vi "ManualPeopleCounting.vi"() -> ()   [LabVIEW 2011]
panel:
  in  "Note 0":string="N"
  in  "0":bool
  in  "Note -3+1":string="N"
  in  "Note +3-1":string="N"
  in  "-3+1":bool
  in  "+3-1":bool
  in  "Note -2+1":string="N"
  in  "Note +2-1":string="N"
  in  "-2+1":bool
  in  "+2-1":bool
  in  "Note -5":string="N"
  in  "- 5":bool
  in  "+5":bool
  in  "Note +5":string="N"
  in  "Note -4":string="N"
  in  "- 4":bool
  in  "+ 4":bool
  in  "Note +4":string="N"
  in  "-999":bool
  in  "Note -999":string="GoOut"
  in  "Note 999":string="N"
  in  "Note -1+1":string="N"
  in  "Note +-1":string="N"
  in  "Note -3":string="N"
  in  "Note +3":string="N"
  in  "Note -2":string="N"
  in  "Note +2":string="N"
  in  "999":bool
  in  "-1+1":bool
  in  "- 3":bool
  in  "+1-1":bool
  in  "+3":bool
  in  "- 2":bool
  in  "+2":bool
  in  "-1":bool
  in  "Note -1":string="N"
  in  "Note +1":string="N"
  in  "+1":bool
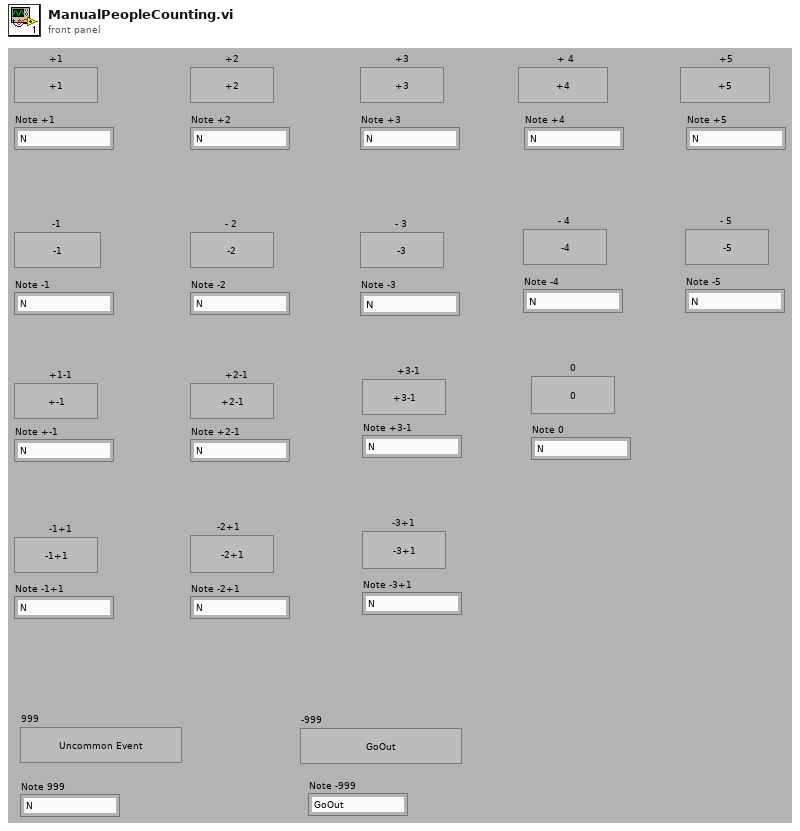
[diagram p1: front panel]
types:
  T1 = enum16{"open", "replace", "create", "open or create", "replace or create", "replace or create with confirmation"}
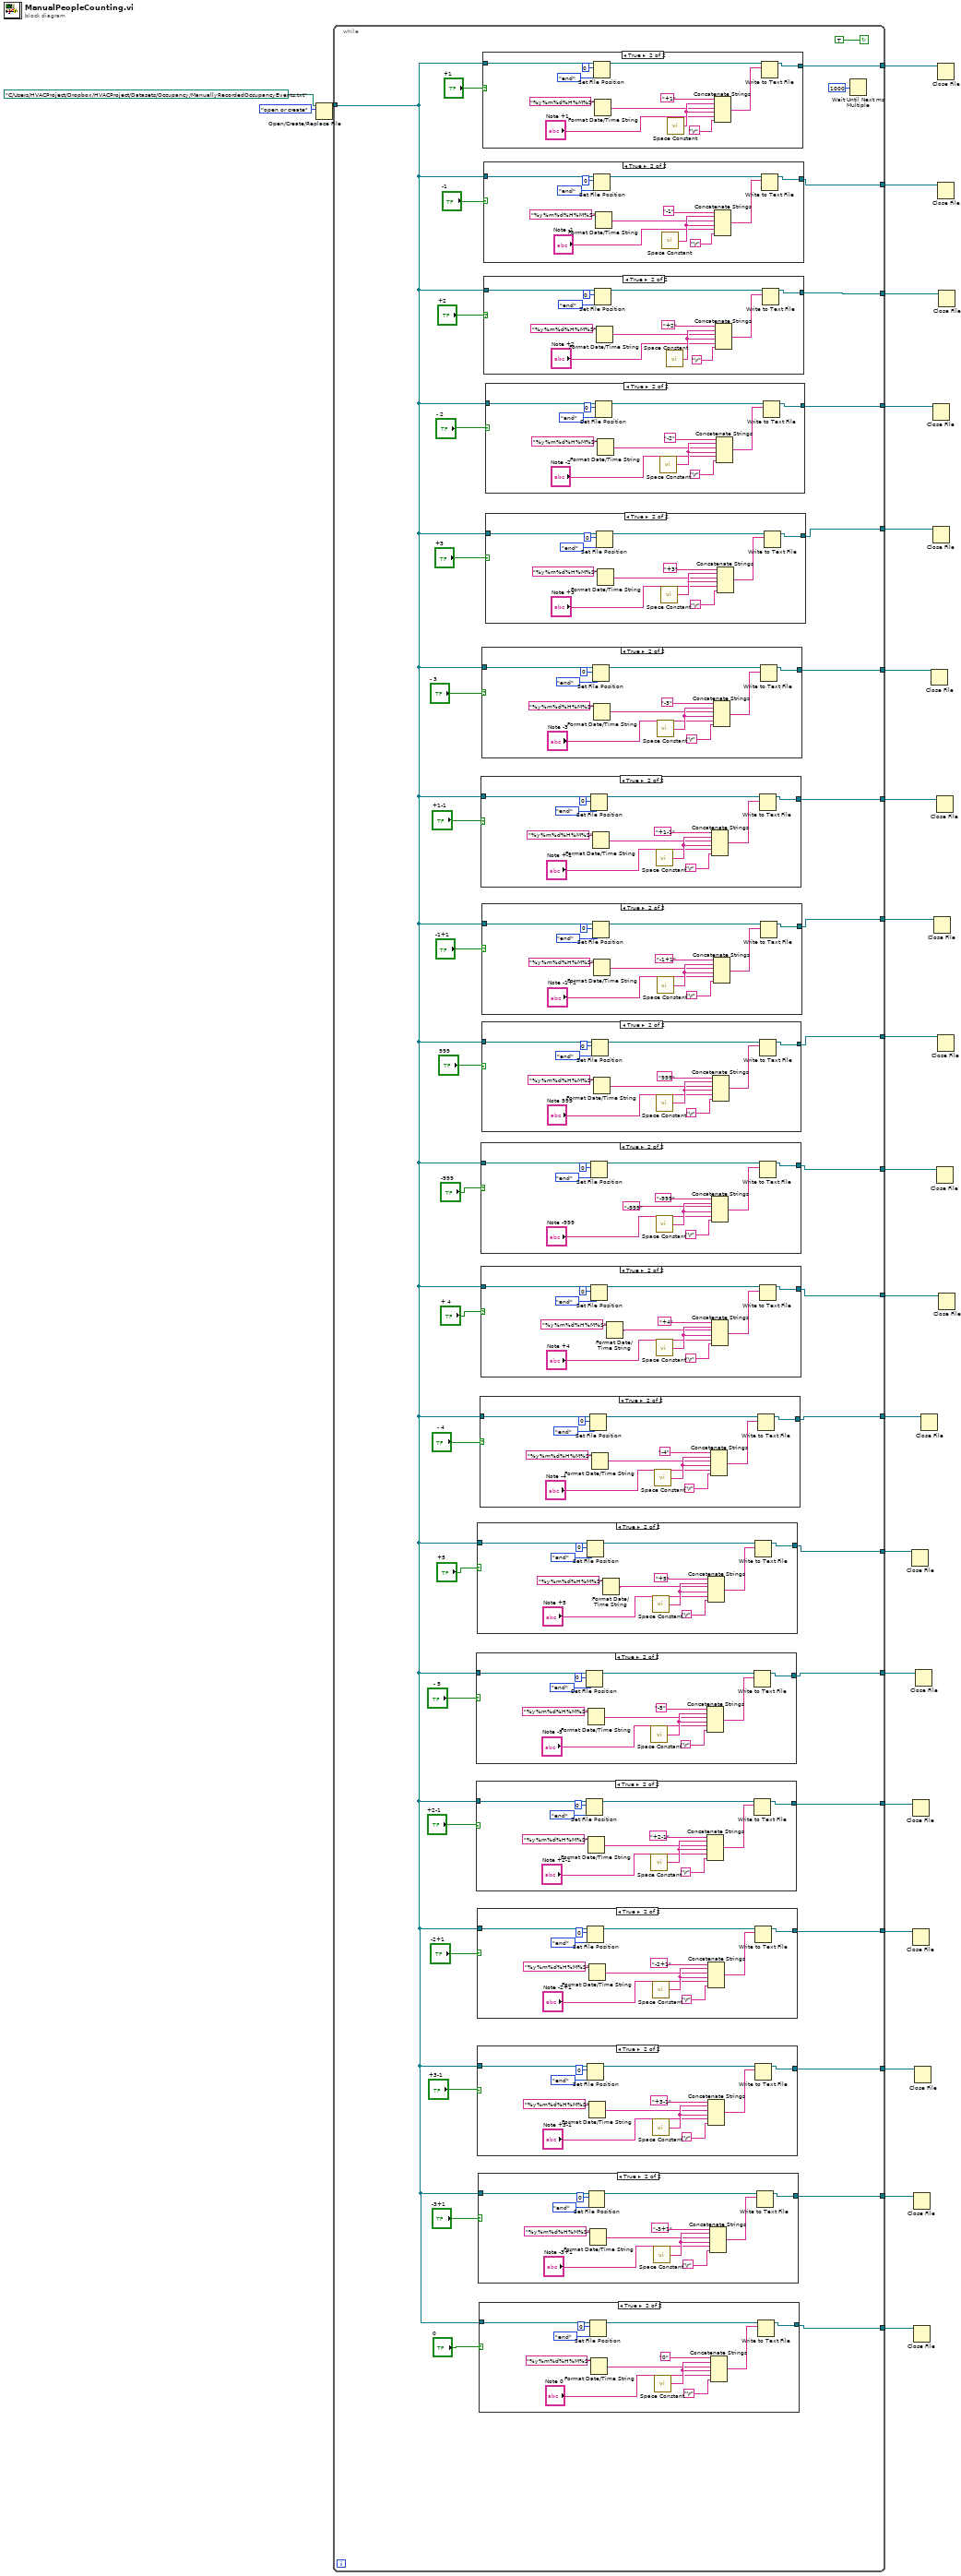
[diagram p0: block diagram]
diagram:
  n1 = Open/Create/Replace File(file path (use dialog)=path "C:/Users/HVACProject/Dropbox/HVACProject/Datasets/Occupancy/ManuallyRecordedOccupancyEvents.txt" ("file (use dialog)"), operation (0:open)=T1."open or create") -> (refnum out=w20:refnum<file>)  [unwired: 4 in, 2 out]
  n2 = while {
    tunnel: w20 -> [w24]
    tunnel: [w59] -> w19
    tunnel: [w58] -> w18
    tunnel: [w56] -> w17
    tunnel: [w54] -> w16
    tunnel: [w52] -> w15
    tunnel: [w50] -> w14
    tunnel: [w48] -> w13
    tunnel: [w46] -> w12
    tunnel: [w44] -> w11
    tunnel: [w43] -> w10
    tunnel: [w40] -> w9
    tunnel: [w38] -> w8
    tunnel: [w35] -> w7
    tunnel: [w34] -> w6
    tunnel: [w31] -> w5
    tunnel: [w30] -> w4
    tunnel: [w27] -> w3
    tunnel: [w26] -> w2
    tunnel: [w23] -> w1
    stop <- TRUE continue-if-true
    n3 = case shown="True" "- 5" {
      tunnel: [w129 w131] -> w35
      tunnel: w24 -> [w129 w141]
      frame False {
      }
      frame True {
        n4 = Set File Position(offset (in bytes) (0)=i64 0, refnum=w141, from (0:start)=enum16{"start", "end", "current"}."end") -> (refnum out=w138:refnum<file>)  [unwired: 1 in, 1 out]
        n5 = Format Date/Time String(time format string (%c)="%y%m%d%H%M%S") -> (date/time string=w133:string)  [unwired: 2 in]
        n6 = call <vilib>:"Space Constant.vi"() -> ("String"=w135:string)
        n7 = Concatenate Strings("-5" ("string"), w135, w133, w135, "Note -5", "\r") -> (w137:string)
        n8 = Write to Text File(file (use dialog)=w138, text=w137) -> (refnum out=w131:refnum<file>)  [unwired: 2 in, 2 out]
      }
    }
    n9 = case shown="True" "+2-1" {
      tunnel: [w116 w118] -> w31
      tunnel: w24 -> [w116 w128]
      frame False {
      }
      frame True {
        n10 = Set File Position(offset (in bytes) (0)=i64 0, refnum=w128, from (0:start)=enum16{"start", "end", "current"}."end") -> (refnum out=w125:refnum<file>)  [unwired: 1 in, 1 out]
        n11 = Format Date/Time String(time format string (%c)="%y%m%d%H%M%S") -> (date/time string=w120:string)  [unwired: 2 in]
        n12 = call <vilib>:"Space Constant.vi"() -> ("String"=w122:string)
        n13 = Concatenate Strings("+2-1" ("string"), w122, w120, w122, "Note +2-1", "\r") -> (w124:string)
        n14 = Write to Text File(file (use dialog)=w125, text=w124) -> (refnum out=w118:refnum<file>)  [unwired: 2 in, 2 out]
      }
    }
    n15 = case shown="True" "+5" {
      tunnel: [w142 w146] -> w34
      tunnel: w24 -> [w142 w154]
      frame False {
      }
      frame True {
        n16 = Set File Position(offset (in bytes) (0)=i64 0, refnum=w154, from (0:start)=enum16{"start", "end", "current"}."end") -> (refnum out=w151:refnum<file>)  [unwired: 1 in, 1 out]
        n17 = Format Date/Time String(time format string (%c)="%y%m%d%H%M%S") -> (date/time string=w143:string)  [unwired: 2 in]
        n18 = call <vilib>:"Space Constant.vi"() -> ("String"=w148:string)
        n19 = Concatenate Strings("+5" ("string"), w148, w143, w148, "Note +5", "\r") -> (w150:string)
        n20 = Write to Text File(file (use dialog)=w151, text=w150) -> (refnum out=w146:refnum<file>)  [unwired: 2 in, 2 out]
      }
    }
    n21 = case shown="True" "-2+1" {
      tunnel: [w103 w105] -> w30
      tunnel: w24 -> [w103 w115]
      frame False {
      }
      frame True {
        n22 = Set File Position(offset (in bytes) (0)=i64 0, refnum=w115, from (0:start)=enum16{"start", "end", "current"}."end") -> (refnum out=w112:refnum<file>)  [unwired: 1 in, 1 out]
        n23 = Format Date/Time String(time format string (%c)="%y%m%d%H%M%S") -> (date/time string=w107:string)  [unwired: 2 in]
        n24 = call <vilib>:"Space Constant.vi"() -> ("String"=w109:string)
        n25 = Concatenate Strings("-2+1" ("string"), w109, w107, w109, "Note -2+1", "\r") -> (w111:string)
        n26 = Write to Text File(file (use dialog)=w112, text=w111) -> (refnum out=w105:refnum<file>)  [unwired: 2 in, 2 out]
      }
    }
    n27 = case shown="True" "+3-1" {
      tunnel: [w90 w92] -> w27
      tunnel: w24 -> [w90 w102]
      frame False {
      }
      frame True {
        n28 = Set File Position(offset (in bytes) (0)=i64 0, refnum=w102, from (0:start)=enum16{"start", "end", "current"}."end") -> (refnum out=w99:refnum<file>)  [unwired: 1 in, 1 out]
        n29 = Format Date/Time String(time format string (%c)="%y%m%d%H%M%S") -> (date/time string=w94:string)  [unwired: 2 in]
        n30 = call <vilib>:"Space Constant.vi"() -> ("String"=w96:string)
        n31 = Concatenate Strings("+3-1" ("string"), w96, w94, w96, "Note +3-1", "\r") -> (w98:string)
        n32 = Write to Text File(file (use dialog)=w99, text=w98) -> (refnum out=w92:refnum<file>)  [unwired: 2 in, 2 out]
      }
    }
    n33 = case shown="True" "-3+1" {
      tunnel: [w77 w79] -> w26
      tunnel: w24 -> [w77 w89]
      frame False {
      }
      frame True {
        n34 = Set File Position(offset (in bytes) (0)=i64 0, refnum=w89, from (0:start)=enum16{"start", "end", "current"}."end") -> (refnum out=w86:refnum<file>)  [unwired: 1 in, 1 out]
        n35 = Format Date/Time String(time format string (%c)="%y%m%d%H%M%S") -> (date/time string=w81:string)  [unwired: 2 in]
        n36 = call <vilib>:"Space Constant.vi"() -> ("String"=w83:string)
        n37 = Concatenate Strings("-3+1" ("string"), w83, w81, w83, "Note -3+1", "\r") -> (w85:string)
        n38 = Write to Text File(file (use dialog)=w86, text=w85) -> (refnum out=w79:refnum<file>)  [unwired: 2 in, 2 out]
      }
    }
    n39 = case shown="True" "0" {
      tunnel: [w64 w66] -> w23
      tunnel: w24 -> [w64 w76]
      frame False {
      }
      frame True {
        n40 = Set File Position(offset (in bytes) (0)=i64 0, refnum=w76, from (0:start)=enum16{"start", "end", "current"}."end") -> (refnum out=w73:refnum<file>)  [unwired: 1 in, 1 out]
        n41 = Format Date/Time String(time format string (%c)="%y%m%d%H%M%S") -> (date/time string=w68:string)  [unwired: 2 in]
        n42 = call <vilib>:"Space Constant.vi"() -> ("String"=w70:string)
        n43 = Concatenate Strings("0" ("string"), w70, w68, w70, "Note 0", "\r") -> (w72:string)
        n44 = Write to Text File(file (use dialog)=w73, text=w72) -> (refnum out=w66:refnum<file>)  [unwired: 2 in, 2 out]
      }
    }
    n45 = case shown="True" "- 4" {
      tunnel: [w155 w157] -> w38
      tunnel: w24 -> [w155 w167]
      frame False {
      }
      frame True {
        n46 = Set File Position(offset (in bytes) (0)=i64 0, refnum=w167, from (0:start)=enum16{"start", "end", "current"}."end") -> (refnum out=w164:refnum<file>)  [unwired: 1 in, 1 out]
        n47 = Format Date/Time String(time format string (%c)="%y%m%d%H%M%S") -> (date/time string=w159:string)  [unwired: 2 in]
        n48 = call <vilib>:"Space Constant.vi"() -> ("String"=w161:string)
        n49 = Concatenate Strings("-4" ("string"), w161, w159, w161, "Note -4", "\r") -> (w163:string)
        n50 = Write to Text File(file (use dialog)=w164, text=w163) -> (refnum out=w157:refnum<file>)  [unwired: 2 in, 2 out]
      }
    }
    n51 = case shown="True" "+1-1" {
      tunnel: [w219 w221] -> w48
      tunnel: w24 -> [w219 w231]
      frame False {
      }
      frame True {
        n52 = Set File Position(offset (in bytes) (0)=i64 0, refnum=w231, from (0:start)=enum16{"start", "end", "current"}."end") -> (refnum out=w228:refnum<file>)  [unwired: 1 in, 1 out]
        n53 = Format Date/Time String(time format string (%c)="%y%m%d%H%M%S") -> (date/time string=w223:string)  [unwired: 2 in]
        n54 = call <vilib>:"Space Constant.vi"() -> ("String"=w225:string)
        n55 = Concatenate Strings("+1-1" ("string"), w225, w223, w225, "Note +-1", "\r") -> (w227:string)
        n56 = Write to Text File(file (use dialog)=w228, text=w227) -> (refnum out=w221:refnum<file>)  [unwired: 2 in, 2 out]
      }
    }
    n57 = case shown="True" "-999" {
      tunnel: [w181 w184] -> w43
      tunnel: w24 -> [w181 w192]
      frame False {
      }
      frame True {
        n58 = Set File Position(offset (in bytes) (0)=i64 0, refnum=w192, from (0:start)=enum16{"start", "end", "current"}."end") -> (refnum out=w189:refnum<file>)  [unwired: 1 in, 1 out]
        n59 = call <vilib>:"Space Constant.vi"() -> ("String"=w186:string)
        n60 = Concatenate Strings("-999" ("string"), w186, "-999" ("string"), w186, "Note -999", "\r") -> (w188:string)
        n61 = Write to Text File(file (use dialog)=w189, text=w188) -> (refnum out=w184:refnum<file>)  [unwired: 2 in, 2 out]
      }
    }
    n62 = case shown="True" "+ 4" {
      tunnel: [w168 w172] -> w40
      tunnel: w24 -> [w168 w180]
      frame False {
      }
      frame True {
        n63 = Set File Position(offset (in bytes) (0)=i64 0, refnum=w180, from (0:start)=enum16{"start", "end", "current"}."end") -> (refnum out=w177:refnum<file>)  [unwired: 1 in, 1 out]
        n64 = Format Date/Time String(time format string (%c)="%y%m%d%H%M%S") -> (date/time string=w169:string)  [unwired: 2 in]
        n65 = call <vilib>:"Space Constant.vi"() -> ("String"=w174:string)
        n66 = Concatenate Strings("+4" ("string"), w174, w169, w174, "Note +4", "\r") -> (w176:string)
        n67 = Write to Text File(file (use dialog)=w177, text=w176) -> (refnum out=w172:refnum<file>)  [unwired: 2 in, 2 out]
      }
    }
    n68 = case shown="True" "999" {
      tunnel: [w193 w195] -> w44
      tunnel: w24 -> [w193 w205]
      frame False {
      }
      frame True {
        n69 = Set File Position(offset (in bytes) (0)=i64 0, refnum=w205, from (0:start)=enum16{"start", "end", "current"}."end") -> (refnum out=w202:refnum<file>)  [unwired: 1 in, 1 out]
        n70 = Format Date/Time String(time format string (%c)="%y%m%d%H%M%S") -> (date/time string=w197:string)  [unwired: 2 in]
        n71 = call <vilib>:"Space Constant.vi"() -> ("String"=w199:string)
        n72 = Concatenate Strings("999" ("string"), w199, w197, w199, "Note 999", "\r") -> (w201:string)
        n73 = Write to Text File(file (use dialog)=w202, text=w201) -> (refnum out=w195:refnum<file>)  [unwired: 2 in, 2 out]
      }
    }
    n74 = case shown="True" "- 3" {
      tunnel: [w232 w234] -> w50
      tunnel: w24 -> [w232 w244]
      frame False {
      }
      frame True {
        n75 = Set File Position(offset (in bytes) (0)=i64 0, refnum=w244, from (0:start)=enum16{"start", "end", "current"}."end") -> (refnum out=w241:refnum<file>)  [unwired: 1 in, 1 out]
        n76 = Format Date/Time String(time format string (%c)="%y%m%d%H%M%S") -> (date/time string=w236:string)  [unwired: 2 in]
        n77 = call <vilib>:"Space Constant.vi"() -> ("String"=w238:string)
        n78 = Concatenate Strings("-3" ("string"), w238, w236, w238, "Note -3", "\r") -> (w240:string)
        n79 = Write to Text File(file (use dialog)=w241, text=w240) -> (refnum out=w234:refnum<file>)  [unwired: 2 in, 2 out]
      }
    }
    n80 = case shown="True" "-1+1" {
      tunnel: [w206 w208] -> w46
      tunnel: w24 -> [w206 w218]
      frame False {
      }
      frame True {
        n81 = Set File Position(offset (in bytes) (0)=i64 0, refnum=w218, from (0:start)=enum16{"start", "end", "current"}."end") -> (refnum out=w215:refnum<file>)  [unwired: 1 in, 1 out]
        n82 = Format Date/Time String(time format string (%c)="%y%m%d%H%M%S") -> (date/time string=w210:string)  [unwired: 2 in]
        n83 = call <vilib>:"Space Constant.vi"() -> ("String"=w212:string)
        n84 = Concatenate Strings("-1+1" ("string"), w212, w210, w212, "Note -1+1", "\r") -> (w214:string)
        n85 = Write to Text File(file (use dialog)=w215, text=w214) -> (refnum out=w208:refnum<file>)  [unwired: 2 in, 2 out]
      }
    }
    n86 = case shown="True" "+1" {
      tunnel: [w297 w299] -> w59
      tunnel: w24 -> [w297 w309]
      frame False {
      }
      frame True {
        n87 = Set File Position(offset (in bytes) (0)=i64 0, refnum=w309, from (0:start)=enum16{"start", "end", "current"}."end") -> (refnum out=w306:refnum<file>)  [unwired: 1 in, 1 out]
        n88 = Format Date/Time String(time format string (%c)="%y%m%d%H%M%S") -> (date/time string=w301:string)  [unwired: 2 in]
        n89 = call <vilib>:"Space Constant.vi"() -> ("String"=w303:string)
        n90 = Concatenate Strings("+1" ("string"), w303, w301, w303, "Note +1", "\r") -> (w305:string)
        n91 = Write to Text File(file (use dialog)=w306, text=w305) -> (refnum out=w299:refnum<file>)  [unwired: 2 in, 2 out]
      }
    }
    n92 = case shown="True" "-1" {
      tunnel: [w284 w286] -> w58
      tunnel: w24 -> [w284 w296]
      frame False {
      }
      frame True {
        n93 = Set File Position(offset (in bytes) (0)=i64 0, refnum=w296, from (0:start)=enum16{"start", "end", "current"}."end") -> (refnum out=w293:refnum<file>)  [unwired: 1 in, 1 out]
        n94 = Format Date/Time String(time format string (%c)="%y%m%d%H%M%S") -> (date/time string=w288:string)  [unwired: 2 in]
        n95 = call <vilib>:"Space Constant.vi"() -> ("String"=w290:string)
        n96 = Concatenate Strings("-1" ("string"), w290, w288, w290, "Note -1", "\r") -> (w292:string)
        n97 = Write to Text File(file (use dialog)=w293, text=w292) -> (refnum out=w286:refnum<file>)  [unwired: 2 in, 2 out]
      }
    }
    n98 = case shown="True" "+2" {
      tunnel: [w271 w273] -> w56
      tunnel: w24 -> [w271 w283]
      frame False {
      }
      frame True {
        n99 = Set File Position(offset (in bytes) (0)=i64 0, refnum=w283, from (0:start)=enum16{"start", "end", "current"}."end") -> (refnum out=w280:refnum<file>)  [unwired: 1 in, 1 out]
        n100 = Format Date/Time String(time format string (%c)="%y%m%d%H%M%S") -> (date/time string=w275:string)  [unwired: 2 in]
        n101 = call <vilib>:"Space Constant.vi"() -> ("String"=w277:string)
        n102 = Concatenate Strings("+2" ("string"), w277, w275, w277, "Note +2", "\r") -> (w279:string)
        n103 = Write to Text File(file (use dialog)=w280, text=w279) -> (refnum out=w273:refnum<file>)  [unwired: 2 in, 2 out]
      }
    }
    n104 = case shown="True" "- 2" {
      tunnel: [w258 w260] -> w54
      tunnel: w24 -> [w258 w270]
      frame False {
      }
      frame True {
        n105 = Set File Position(offset (in bytes) (0)=i64 0, refnum=w270, from (0:start)=enum16{"start", "end", "current"}."end") -> (refnum out=w267:refnum<file>)  [unwired: 1 in, 1 out]
        n106 = Format Date/Time String(time format string (%c)="%y%m%d%H%M%S") -> (date/time string=w262:string)  [unwired: 2 in]
        n107 = call <vilib>:"Space Constant.vi"() -> ("String"=w264:string)
        n108 = Concatenate Strings("-2" ("string"), w264, w262, w264, "Note -2", "\r") -> (w266:string)
        n109 = Write to Text File(file (use dialog)=w267, text=w266) -> (refnum out=w260:refnum<file>)  [unwired: 2 in, 2 out]
      }
    }
    n110 = case shown="True" "+3" {
      tunnel: [w245 w247] -> w52
      tunnel: w24 -> [w245 w257]
      frame False {
      }
      frame True {
        n111 = Set File Position(offset (in bytes) (0)=i64 0, refnum=w257, from (0:start)=enum16{"start", "end", "current"}."end") -> (refnum out=w254:refnum<file>)  [unwired: 1 in, 1 out]
        n112 = Format Date/Time String(time format string (%c)="%y%m%d%H%M%S") -> (date/time string=w249:string)  [unwired: 2 in]
        n113 = call <vilib>:"Space Constant.vi"() -> ("String"=w251:string)
        n114 = Concatenate Strings("+3" ("string"), w251, w249, w251, "Note +3", "\r") -> (w253:string)
        n115 = Write to Text File(file (use dialog)=w254, text=w253) -> (refnum out=w247:refnum<file>)  [unwired: 2 in, 2 out]
      }
    }
    n116 = Wait Until Next ms Multiple(millisecond multiple=u32 1000) -> ()  [unwired: 1 out]
  }
  n117 = Close File(refnum=w6) -> ()  [unwired: 1 in, 2 out]
  n118 = Close File(refnum=w5) -> ()  [unwired: 1 in, 2 out]
  n119 = Close File(refnum=w4) -> ()  [unwired: 1 in, 2 out]
  n120 = Close File(refnum=w2) -> ()  [unwired: 1 in, 2 out]
  n121 = Close File(refnum=w1) -> ()  [unwired: 1 in, 2 out]
  n122 = Close File(refnum=w3) -> ()  [unwired: 1 in, 2 out]
  n123 = Close File(refnum=w7) -> ()  [unwired: 1 in, 2 out]
  n124 = Close File(refnum=w8) -> ()  [unwired: 1 in, 2 out]
  n125 = Close File(refnum=w14) -> ()  [unwired: 1 in, 2 out]
  n126 = Close File(refnum=w16) -> ()  [unwired: 1 in, 2 out]
  n127 = Close File(refnum=w15) -> ()  [unwired: 1 in, 2 out]
  n128 = Close File(refnum=w12) -> ()  [unwired: 1 in, 2 out]
  n129 = Close File(refnum=w13) -> ()  [unwired: 1 in, 2 out]
  n130 = Close File(refnum=w10) -> ()  [unwired: 1 in, 2 out]
  n131 = Close File(refnum=w11) -> ()  [unwired: 1 in, 2 out]
  n132 = Close File(refnum=w19) -> ()  [unwired: 1 in, 2 out]
  n133 = Close File(refnum=w18) -> ()  [unwired: 1 in, 2 out]
  n134 = Close File(refnum=w17) -> ()  [unwired: 1 in, 2 out]
  n135 = Close File(refnum=w9) -> ()  [unwired: 1 in, 2 out]
